vi "Query Peak Over.vi"(8 "error in (no error)":errorcluster, 11 "VISA resource name":refnum<visa-resource-name>) -> (0 "error out":errorcluster, 1 "Peak Over List":bool[](array[boolean]), 2 "Peak Over":i32, 3 "VISA resource name out":refnum<visa-resource-name>)   [LabVIEW 2016, in "Yokogawa WT300 Series.lvlib"]
doc: "Queries the peak over-range information."
uses:
  Yokogawa WT300 Series.lvlib
panel:
  # "U1"
  # "I1"
  # "U2"
  # "I2"
  # "U3"
  # "I3"
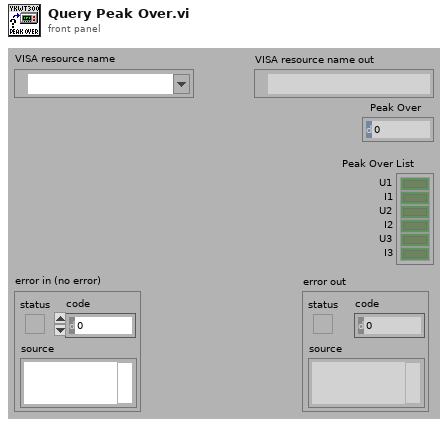
[diagram p1: front panel]
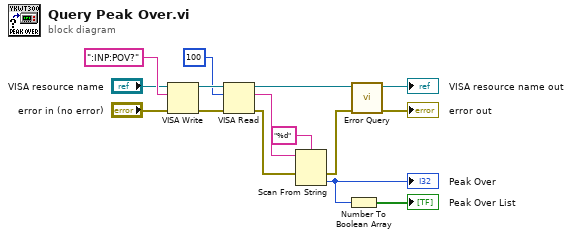
[diagram p0: block diagram]
diagram:
  n1 = VISA Write ("VISA書き込み")(VISA resource name="VISA resource name", write buffer=":INP:POV?", error in (no error)="error in (no error)") -> (VISA resource name out=w14:refnum<visa-resource-name>, error out=w15:errorcluster)  [unwired: 1 out]
  n2 = VISA Read ("VISA読み取り")(VISA resource name=w14, byte count=u32 100, error in (no error)=w15) -> (VISA resource name out=w6:refnum<visa-resource-name>, read buffer=w8:string, error out=w7:errorcluster)  [unwired: 1 out]
  n3 = Scan From String ("文字列からスキャン")(format string="%d", input string=w8, error in=w7) -> (error out=w4:errorcluster, output 1=w1:i32)  [unwired: 2 in, 2 out]
  "Peak Over" <- w1
  n4 = Number To Boolean Array(number=w1) -> (Boolean array=→"Peak Over List":bool[])
  n5 = call "Error Query.vi"("error in (no error)"=w4, "VISA resource name"=w6) -> ("error out"=→"error out":errorcluster, "VISA resource name out"=→"VISA resource name out":refnum<visa-resource-name>)  [unwired: 6 in, 2 out]
